vi "Generate Standard Waveform (SubVI).vi"(0 "VISA Refnum in":refnum<visa-resource-name>, 1 "Enable Output (T: Enable)":bool=TRUE, 2 "Envelope Decay Time":dbl=50.0, 5 "Phase Before Trigger":dbl=0.15 format="%#_13g", 7 "time (us)":dbl, 9 "Frequency (1000 Hz)":dbl=1000.0, 11 "t before":dbl=2.0 format="%#_13g", 14 "Amplitude (1 Vpp)":dbl=1.0) -> ()   [LabVIEW 2016]
uses:
  Tektronix AFG 1000 Series.lvlib
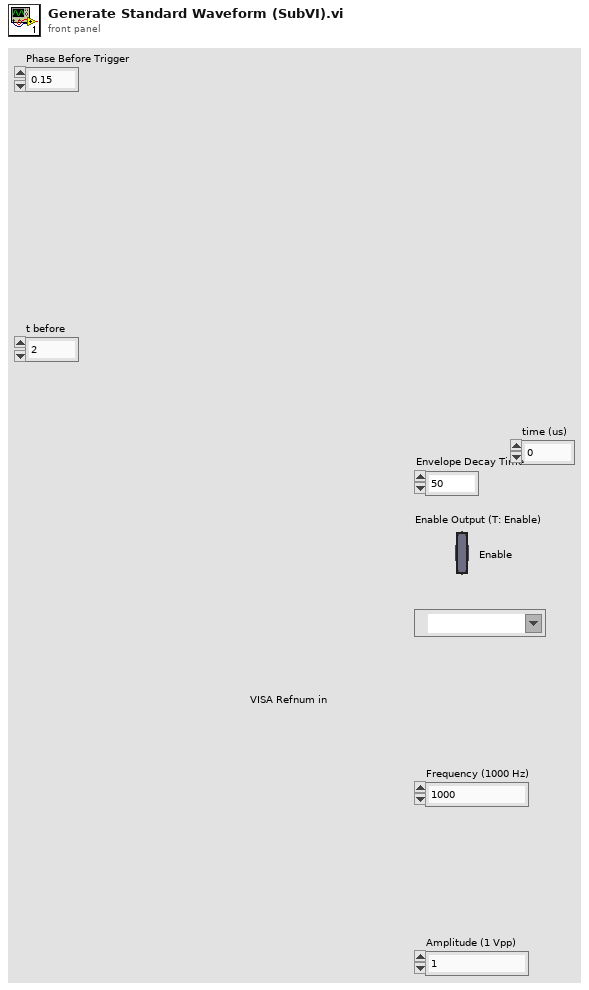
[diagram p1: front panel]
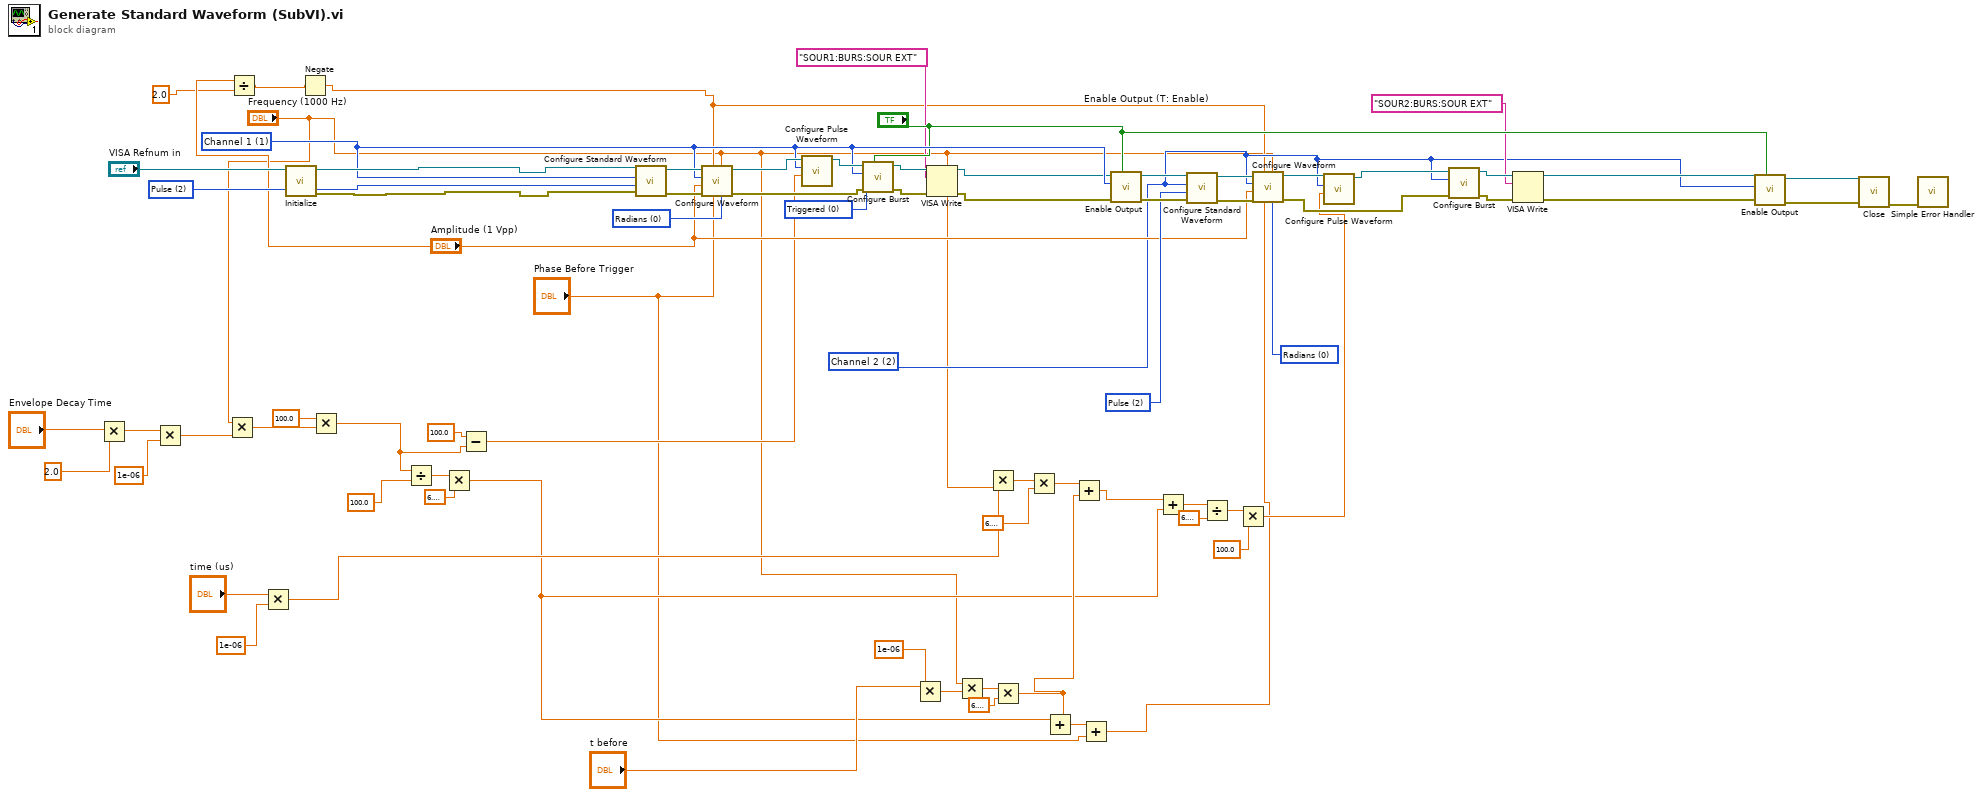
[diagram p0: block diagram]
diagram:
  w40 = u16 0 items=["Triggered", "Gated"] ("Burst Mode (0: Triggered)")
  w64 = u16 0 items=["Radians", "Degrees"] ("Phase Unit (0: Radian)")
  w67 = u16 2 items=["Sine", "Square", "Pulse", "Ramp", "Noise"] ("Waveform Function (0: Sine)")
  w41 = u16 1 items=["Channel 1"=1, "Channel 2"=2] ("Channel (1 Channel 1)")
  w26 = u16 2 items=["Channel 1"=1, "Channel 2"=2] ("Channel (1 Channel 1)")
  w68 = u16 2 items=["Sine", "Square", "Pulse", "Ramp", "Noise"] ("Waveform Function (0: Sine)")
  w72 = u16 0 items=["Radians", "Degrees"] ("Phase Unit (0: Radian)")
  n1 = Multiply(x="Envelope Decay Time", y=2.0) -> (x*y=w10:dbl)
  n2 = Multiply(x=w10, y=1e-06) -> (x*y=w8:dbl)
  n3 = Multiply(x="Frequency (1000 Hz)", y=w8) -> (x*y=w7:dbl)
  n4 = Divide(x="Amplitude (1 Vpp)", y=2.0) -> (x/y=w25:dbl)
  n5 = Multiply(x="time (us)", y=1e-06) -> (x*y=w56:dbl)
  n6 = call "Initialize.vi"("VISA resource name"="VISA Refnum in") -> ("error out"=w44:errorcluster, "VISA resource name out"=w45:refnum<visa-resource-name>)  [unwired: 9 in]
  n7 = Negate(x=w25) -> (-x=w24:dbl)
  n8 = Multiply(x=100.0, y=w7) -> (x*y=w5:dbl)
  n9 = Divide(x=w5, y=100.0) -> (x/y=w52:dbl)
  n10 = Multiply(x=w52, y=6.283185307179586) -> (x*y=w13:dbl)
  n11 = Subtract(x=100.0, y=w5) -> (x-y=w22:dbl)
  n12 = call "Configure Standard Waveform.vi"("error in (no error)"=w44, "Waveform Function (0: Sine)"=w68, "Channel (1 Channel 1)"=w41, "VISA resource name"=w45) -> ("error out"=w74:errorcluster, "VISA resource name out"=w73:refnum<visa-resource-name>)  [unwired: 6 in]
  n13 = call "Configure Waveform.vi"("Phase Unit (0: Radian)"=w72, "Frequency (1000 Hz)"="Frequency (1000 Hz)", "Phase (0)"="Phase Before Trigger", "DC Offset (0.00 V)"=w24, "error in (no error)"=w74, "Amplitude (1 Vpp)"="Amplitude (1 Vpp)", "Channel (1 Channel 1)"=w41, "VISA resource name"=w73) -> ("error out"=w42:errorcluster, "VISA resource name out"=w71:refnum<visa-resource-name>)  [unwired: 2 in]
  n14 = call "Configure Pulse Waveform.vi"("Duty Cycle (50%)"=w22, "Channel (1: Channel 1)"=w41, "VISA resource name"=w71) -> ("VISA resource name out"=w43:refnum<visa-resource-name>)  [unwired: 7 in, 1 out]
  n15 = call "Configure Burst.vi"("Enable Burst (T: Enable)"="Enable Output (T: Enable)", "error in (no error)"=w42, "Burst Mode (0: Triggered)"=w40, "Channel (1 Channel 1)"=w41, "VISA resource name"=w43) -> ("error out"=w37:errorcluster, "VISA resource name out"=w39:refnum<visa-resource-name>)  [unwired: 5 in]
  n16 = Multiply(x="t before", y=1e-06) -> (x*y=w48:dbl)
  n17 = VISA Write(VISA resource name=w39, write buffer="SOUR1:BURS:SOUR EXT", error in (no error)=w37) -> (VISA resource name out=w36:refnum<visa-resource-name>, error out=w35:errorcluster)  [unwired: 1 out]
  n18 = Multiply(x="Frequency (1000 Hz)", y=w48) -> (x*y=w47:dbl)
  n19 = Multiply(x=w56, y="Frequency (1000 Hz)") -> (x*y=w55:dbl)
  n20 = Multiply(x=w47, y=6.283185307179586) -> (x*y=w14:dbl)
  n21 = Multiply(x=w55, y=6.283185307179586) -> (x*y=w21:dbl)
  n22 = Add(x=w13, y=w14) -> (x+y=w3:dbl)
  n23 = Add(x=w21, y=w14) -> (x+y=w20:dbl)
  n24 = Add(x=w3, y="Phase Before Trigger") -> (x+y=w1:dbl)
  n25 = call "Enable Output.vi"("Enable Output (T: Enable)"="Enable Output (T: Enable)", "error in (no error)"=w35, "Channel (1: Channel 1)"=w41, "VISA resource name"=w36) -> ("error out"=w69:errorcluster, "VISA resource name out"=w70:refnum<visa-resource-name>)  [unwired: 6 in]
  n26 = Add(x=w20, y=w13) -> (x+y=w19:dbl)
  n27 = call "Configure Standard Waveform.vi"("error in (no error)"=w69, "Waveform Function (0: Sine)"=w67, "Channel (1 Channel 1)"=w26, "VISA resource name"=w70) -> ("error out"=w65:errorcluster, "VISA resource name out"=w66:refnum<visa-resource-name>)  [unwired: 6 in]
  n28 = Divide(x=w19, y=6.283185307179586) -> (x/y=w17:dbl)
  n29 = Multiply(x=w17, y=100.0) -> (x*y=w15:dbl)
  n30 = call "Configure Waveform.vi"("Phase Unit (0: Radian)"=w64, "Frequency (1000 Hz)"="Frequency (1000 Hz)", "Phase (0)"=w1, "DC Offset (0.00 V)"=w24, "error in (no error)"=w65, "Amplitude (1 Vpp)"="Amplitude (1 Vpp)", "Channel (1 Channel 1)"=w26, "VISA resource name"=w66) -> ("error out"=w33:errorcluster, "VISA resource name out"=w63:refnum<visa-resource-name>)  [unwired: 2 in]
  n31 = call "Configure Pulse Waveform.vi"("Duty Cycle (50%)"=w15, "Channel (1: Channel 1)"=w26, "VISA resource name"=w63) -> ("VISA resource name out"=w27:refnum<visa-resource-name>)  [unwired: 7 in, 1 out]
  n32 = call "Configure Burst.vi"("error in (no error)"=w33, "Channel (1 Channel 1)"=w26, "VISA resource name"=w27) -> ("error out"=w32:errorcluster, "VISA resource name out"=w29:refnum<visa-resource-name>)  [unwired: 7 in]
  n33 = VISA Write(VISA resource name=w29, write buffer="SOUR2:BURS:SOUR EXT", error in (no error)=w32) -> (VISA resource name out=w30:refnum<visa-resource-name>, error out=w31:errorcluster)  [unwired: 1 out]
  n34 = call "Enable Output.vi"("Enable Output (T: Enable)"="Enable Output (T: Enable)", "error in (no error)"=w31, "Channel (1: Channel 1)"=w26, "VISA resource name"=w30) -> ("error out"=w61:errorcluster, "VISA resource name out"=w62:refnum<visa-resource-name>)  [unwired: 6 in]
  n35 = call "Close.vi"("error in (no error)"=w61, "VISA resource name"=w62) -> ("error out"=w76:errorcluster)  [unwired: 9 in]
  n36 = call <vilib>:"Simple Error Handler.vi"("error in (no error)"=w76) -> ()  [unwired: 4 in, 5 out]
